vi "Level Sensors Calibrator.vi"(5 "Data in":T1) -> (2 "Data out":T1)   [LabVIEW 2018]
doc: "This VI calibrates sensors values."
panel:
  in  "y 2":dbl[](array[numeric])=[0.0, 0.0, 0.0, 0.0]
  in  "y":dbl[](array[numeric])=[2.75, 2.55, 3.0, 2.6]
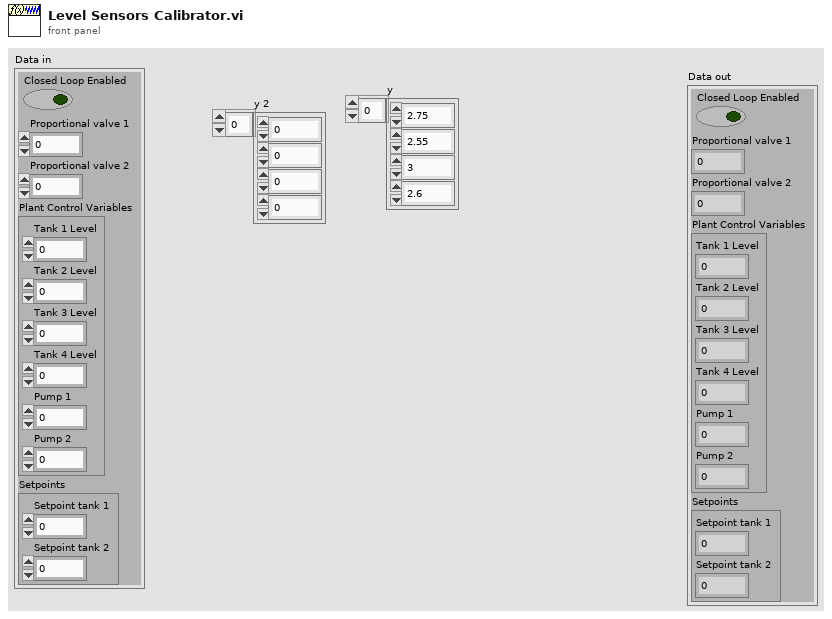
[diagram p1: front panel]
types:
  T1 = cluster{"Closed Loop Enabled":bool, "Proportional valve 1":dbl, "Proportional valve 2":dbl, "Plant Control Variables":cluster{"Tank 1 Level":dbl, "Tank 2 Level":dbl, "Tank 3 Level":dbl, "Tank 4 Level":dbl, "Pump 1":dbl, "Pump 2":dbl}, "Setpoints":cluster{"Setpoint tank 1":dbl, "Setpoint tank 2":dbl}}
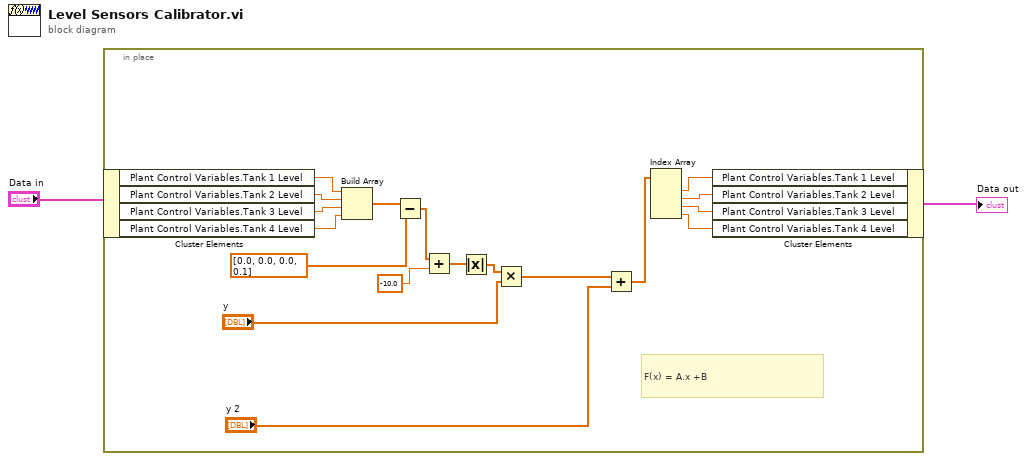
[diagram p0: block diagram]
diagram:
  n1 = in-place {
    # "F(x) = A.x +B"
    n2 = in-place-cluster #1("Data in") -> ("Plant Control Variables.Tank 1 Level"=w17:dbl, "Plant Control Variables.Tank 2 Level"=w16:dbl, "Plant Control Variables.Tank 3 Level"=w15:dbl, "Plant Control Variables.Tank 4 Level"=w14:dbl)
    n3 = Build Array(w17, w16, w15, w14) -> (w5:dbl[])
    n4 = Subtract(x=w5, y=dbl[] [0.0, 0.0, 0.0, 0.1]) -> (x-y=w4:dbl[])
    n5 = Add(x=w4, y=-10.0) -> (x+y=w8:dbl[])
    n6 = Absolute Value(x=w8) -> (abs(x)=w7:dbl[])
    n7 = Multiply(x=w7, y="y") -> (x*y=w6:dbl[])
    n8 = Add(x=w6, y="y 2") -> (x+y=w12:dbl[])
    n9 = Index Array(array=w12) -> (element #1=w13:dbl, element #2=w10:dbl, element #3=w9:dbl, element #4=w11:dbl)  [unwired: 4 in]
    n10 = in-place-cluster #1("Plant Control Variables.Tank 1 Level"=w13, "Plant Control Variables.Tank 2 Level"=w10, "Plant Control Variables.Tank 3 Level"=w9, "Plant Control Variables.Tank 4 Level"=w11) -> (→"Data out":T1)
  }
